vi "Close.vi"(8 "Error In":errorcluster, 11 "Initialization Data":variant) -> (0 "Error Out":errorcluster)   [LabVIEW 2012, in "CS++MessageLogger.lvlib"]
doc: "Close the central message logger."
uses:
  CS++MessageLogger.lvlib
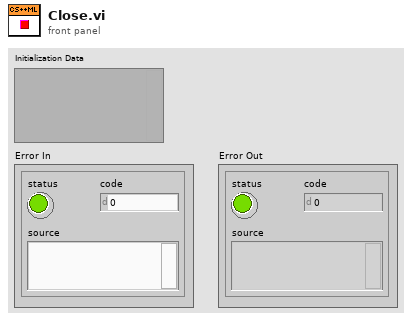
[diagram p1: front panel]
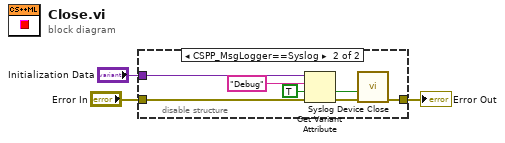
[diagram p0: block diagram]
diagram:
  n1 = disable-structure shown="CSPP_MsgLogger==Syslog" {
    disable-tunnel: "Error In" -> [w4 w9]
    disable-tunnel: [w4 w5] -> w2
    disable-tunnel: "Initialization Data" -> [_ w8]
    frame condition #0 {
    }
    frame condition #1 (active) {
      n2 = Get Variant Attribute(Variant=w8, name="Debug", default value (empty Variant)=TRUE, error in=w9) -> (value=w6:bool, error out=w7:errorcluster)  [unwired: 2 out]
      n3 = call <userlib>:"Syslog Device Close.vi"("error in (no error)"=w7, "Send debug message (T)"=w6) -> ("error out"=w5:errorcluster)  [unwired: 9 in]
    }
  }
  "Error Out" <- w2
